vi "Wait for Message Array.vi"(1 "gui notification":string, 2 "last state":string, 3 "cases to ignore":string[](array[string]), 4 "acquisition state array":string[](array[string])) -> (0 "wait for message?":bool)   [LabVIEW 2020]
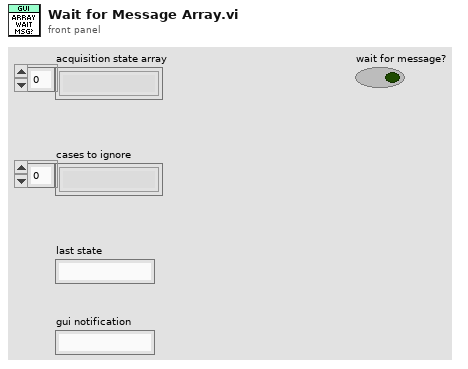
[diagram p1: front panel]
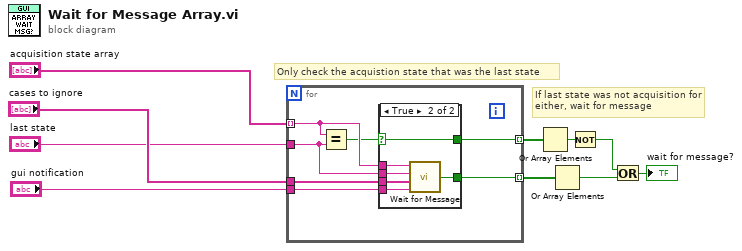
[diagram p0: block diagram]
diagram:
  # "If last state was not acquisition for either, wait for message"
  # "Only check the acquistion state that was the last state"
  n1 = for {
    tunnel: [w17] -> w6 mode=indexing
    tunnel: "last state" -> [w13]
    tunnel: "gui notification" -> [w16]
    tunnel: "cases to ignore" -> [w15]
    tunnel: "acquisition state array" -> [w14] mode=indexing
    tunnel: [w11] -> w5 mode=indexing
    n2 = Equal?(x=w14, y=w13) -> (x = y?=w12:bool)
    n3 = case shown="True" w12 {
      selector: w12 -> [w18 w19]
      tunnel: [w18 w24] -> w17
      tunnel: w16 -> [_ w23]
      tunnel: w15 -> [_ w22]
      tunnel: w14 -> [_ w21]
      tunnel: w13 -> [_ w20]
      tunnel: [w18 w19] -> w11
      frame False {
      }
      frame True {
        n4 = call "Wait for Message.vi"("gui notification"=w23, "cases to ignore"=w22, "last state"=w20, "acquisition state name"=w21) -> ("wait for notification?"=w24:bool)
      }
    }
  }
  n5 = Or Array Elements(Boolean array=w5) -> (logical OR=w4:bool)
  n6 = Or Array Elements(Boolean array=w6) -> (logical OR=w1:bool)
  n7 = Not(x=w4) -> (.not. x?=w2:bool)
  n8 = Or(x=w2, y=w1) -> (x .or. y?=→"wait for message?":bool)
